vi "ConvertScanListToChannels.vi"(11 "Scan List":string) -> (3 "Channels":bool[](array[boolean]))   [LabVIEW 2012]
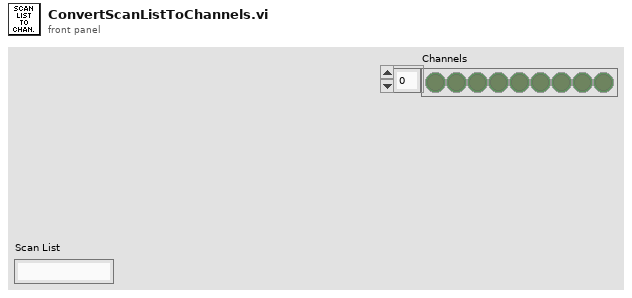
[diagram p1: front panel]
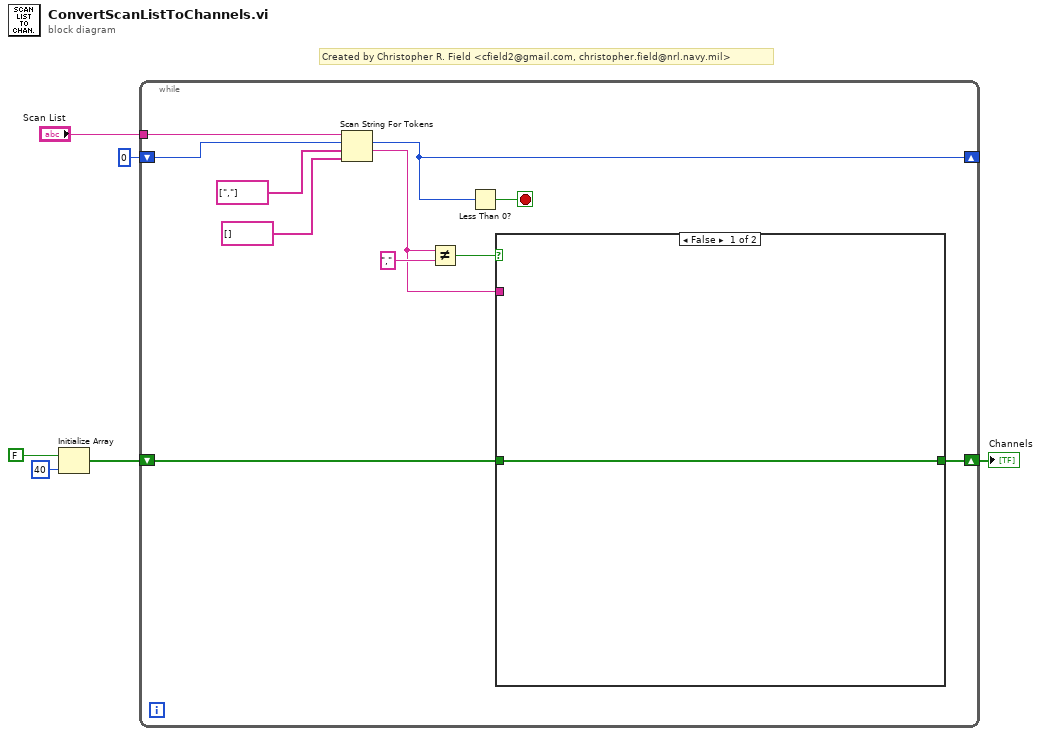
[diagram p0: block diagram]
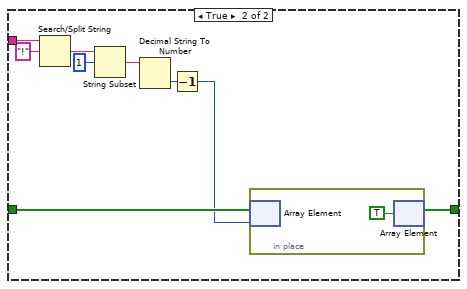
[diagram p2: hidden frame]
diagram:
  # "Created by Christopher R. Field <cfield2@gmail.com, christopher.field@nrl.navy.mil>"
  n1 = Initialize Array(FALSE, 40 ("dimension size")) -> (w2:bool[])
  n2 = while {
    tunnel: "Scan List" -> [w17]
    shift-right: [w12] -> _
    shift-left: 0 -> [w14]
    shift-right: [w7] -> w1
    shift-left: w2 -> [w8]
    stop <- w13 stop-if-true
    n3 = Scan String For Tokens(6:string[] [] ("delimiters (\\s,\\t,\\r,\\n)"), 7:string[] [","] ("operators (none)"), 8:w14, 9:w17) -> (1:w9:string, 2:w12:i32)  [unwired: 2 in, 2 out]
    n4 = Not Equal?(x=w9, y=",") -> (x != y?=w10:bool)
    n5 = Less Than 0?(x=w12) -> (x < 0?=w13:bool)
    n6 = case shown="False" w10 {
      tunnel: w9 -> [_ w27]
      tunnel: w8 -> [w18 w21]
      tunnel: [w18 w19] -> w7
      frame False {
      }
      frame True {
        n7 = Search/Split String(string=w27, search string/char (-)="!") -> (match + rest of string=w25:string)  [unwired: 1 in, 2 out]
        n8 = String Subset(string=w25, offset (0)=1) -> (substring=w23:string)  [unwired: 1 in]
        n9 = Decimal String To Number(string=w23) -> (number=w22:i32)  [unwired: 2 in, 1 out]
        n10 = Decrement(x=w22) -> (x-1=w20:i32)
        n11 = in-place {
          n12 = in-place-array #1(w21, w20) -> ()  [unwired: 1 out]
          n13 = in-place-array #1(TRUE ("element")) -> (w19:bool[])  [unwired: 1 out]
        }
      }
    }
  }
  "Channels" <- w1
